vi "E441X_PM_Read_Measurement.vi"(0 "VISA session":refnum<visa-resource-name>, 1 "Measurement (1)":i32=1, 5 "Measuring Function (0: Single)":i32(ring) items=["Single", "Single Relative", "Difference", "Difference Relative", "Ratio", "Ratio Relative"], 11 "error in (no error)":errorcluster {"code" format="%.0x"}) -> (4 "dup VISA session":refnum<visa-resource-name>, 8 "Measured Value":dbl format="%^.2e", 15 "error out":errorcluster {"code" format="%.0x"})   [LabVIEW 2015]
doc: "This VI initiates the measurement and returns the measured value."
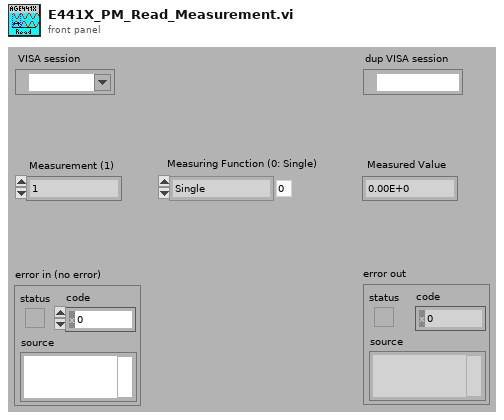
[diagram p1: front panel]
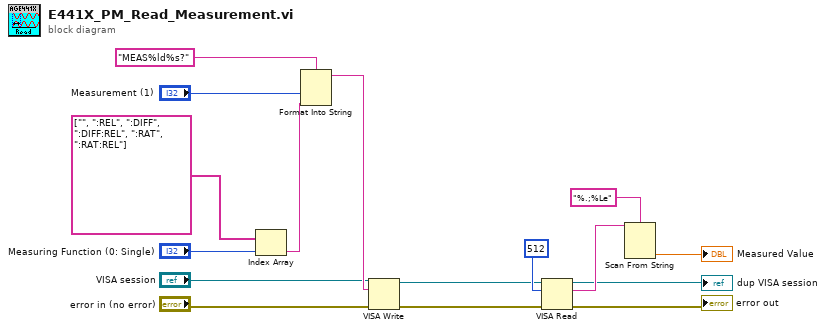
[diagram p0: block diagram]
diagram:
  n1 = Index Array(array=string[] ["", ":REL", ":DIFF", ":DIFF:REL", ":RAT", ":RAT:REL"], index="Measuring Function (0: Single)") -> (element=w13:string)
  n2 = Format Into String(format string="MEAS%ld%s?", "Measurement (1)", w13) -> (resulting string=w12:string)  [unwired: 2 in, 1 out]
  n3 = VISA Write(VISA resource name="VISA session", write buffer=w12, error in (no error)="error in (no error)") -> (VISA resource name out=w2:refnum<visa-resource-name>, error out=w1:errorcluster)  [unwired: 1 out]
  n4 = VISA Read(VISA resource name=w2, byte count=u32 512 ("byte count (0)"), error in (no error)=w1) -> (VISA resource name out=→"dup VISA session":refnum<visa-resource-name>, read buffer=w11:string, error out=→"error out":errorcluster)  [unwired: 1 out]
  n5 = Scan From String(format string="%.;%Le", input string=w11) -> (output 1=→"Measured Value":dbl)  [unwired: 3 in, 3 out]
